vi "Configure PRBS Waveform.vi"(0 "VISA resource name":refnum<visa-resource-name>, 1 "Amplitude (4 Vpp)":dbl=4.0, 2 "Offset (0.00 V)":dbl min=-10.0 max=10.0, 5 "Channel (1: 1)":u16(ring)=1 items=["Channel 1"=1, "Channel 2"=2], 7 "Length (3)":u16=3, 9 "Bit Rate (1000 bits/second)":dbl=1000.0, 11 "error in (no error)":errorcluster, 12 "Edge Time (10 ns)":dbl=1e-08) -> (4 "VISA resource name out":refnum<visa-resource-name>, 15 "error out":errorcluster)   [LabVIEW 2023, in "Siglent SDG X Series.lvlib"]
doc: "Configures PRBS waveform and parameters.\n\nNote:\nThis VI only supports SDG6000X series."
uses:
  Siglent SDG X Series.lvlib
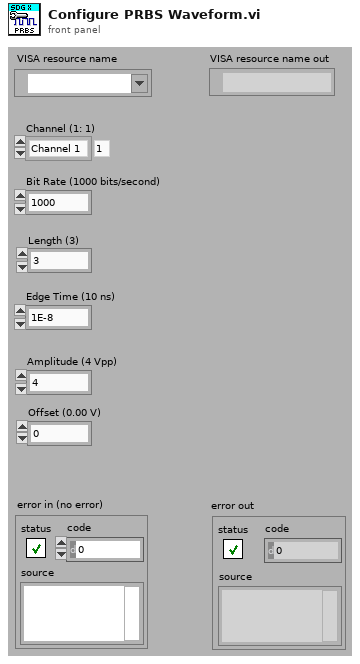
[diagram p1: front panel]
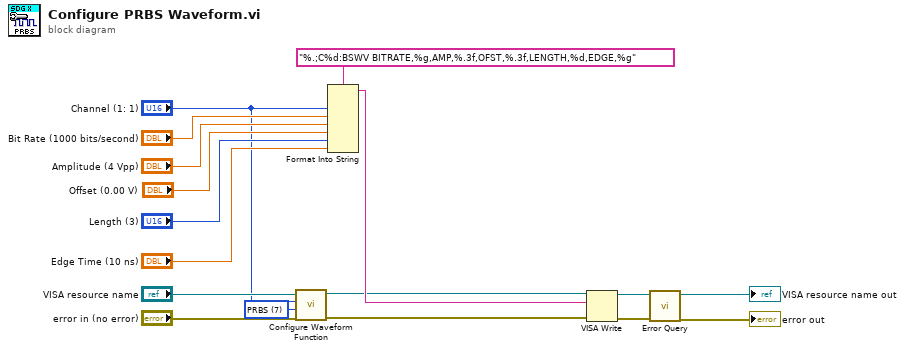
[diagram p0: block diagram]
diagram:
  w3 = u16 7 items=["Sine", "Square", "Ramp", "DC", "Pulse", "Arb", "Noise", "PRBS", "IQ"] ("Waveform Function (0: Sine)")
  n1 = call "Configure Waveform Function.vi"("error in (no error)"="error in (no error)", "Waveform Function (0: Sine)"=w3, "Channel (1:Channel 1)"="Channel (1: 1)", "VISA resource name"="VISA resource name") -> ("error out"=w2:errorcluster, "VISA resource name out"=w1:refnum<visa-resource-name>)  [unwired: 6 in]
  n2 = Format Into String(format string="%.;C%d:BSWV BITRATE,%g,AMP,%.3f,OFST,%.3f,LENGTH,%d,EDGE,%g", "Channel (1: 1)", "Bit Rate (1000 bits/second)", "Amplitude (4 Vpp)", "Offset (0.00 V)", "Length (3)", "Edge Time (10 ns)") -> (resulting string=w7:string)  [unwired: 2 in, 1 out]
  n3 = VISA Write(VISA resource name=w1, write buffer=w7, error in (no error)=w2) -> (VISA resource name out=w17:refnum<visa-resource-name>, error out=w16:errorcluster)  [unwired: 1 out]
  n4 = call "Error Query.vi"("error in (no error)"=w16, "VISA resource name"=w17) -> ("error out"=→"error out":errorcluster, "VISA resource name out"=→"VISA resource name out":refnum<visa-resource-name>)  [unwired: 6 in, 2 out]
